vi "Get Enum Strings.vi"(8 "error in (no error)":errorcluster, 9 "Units":bool, 10 "Type":bool) -> (0 "error out":errorcluster, 1 "Units":cluster{"String":string, "Value":u16}[](array[cluster]), 2 "Type":cluster{"String":string, "Value":u16}[](array[cluster]))   [LabVIEW 2017, in "Modules.lvlib" / "9213.lvclass"]
uses:
  9213.lvclass
  Thermocouple Type.ctl
  Measurement Units.ctl
panel:
  out "Measurement Units":T1 items=["Raw Volts", "Degrees Kelvin", "Degrees Celsius", "Degrees Fahrenheit", "Degrees Rankine"]
  out "Thermocouple Type":T2 items=["J", "K", "T", "E", "R", "S", "N", "B"]
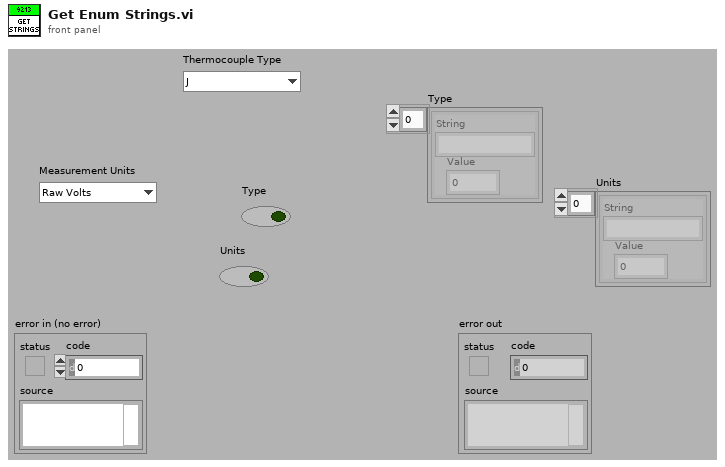
[diagram p1: front panel]
types:
  T1 = typedef "Modules.lvlib/9213.lvclass/Measurement Units.ctl" = u8
  T2 = typedef "Modules.lvlib/9213.lvclass/Thermocouple Type.ctl" = u8
  T3 = typedef "LVStringsAndValuesArrayTypeDef_U8.ctl" = cluster{"String":string, "Value":u8}[]
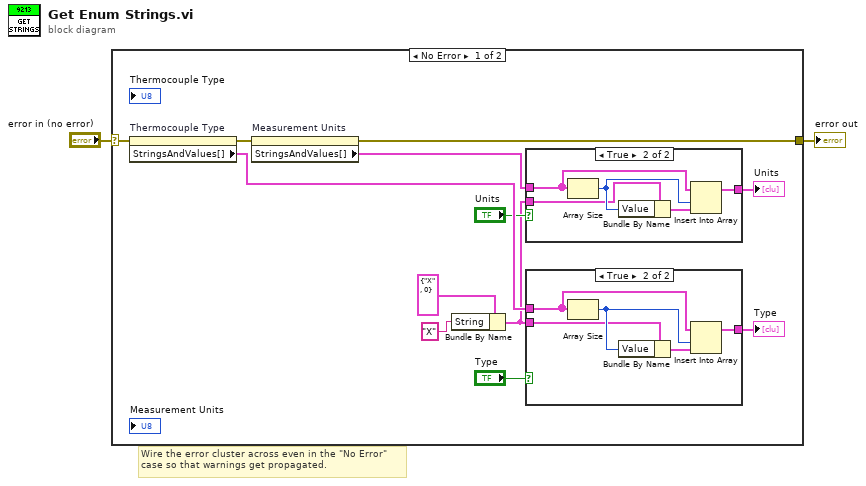
[diagram p0: block diagram]
diagram:
  # "Wire the error cluster across even in the \"No Error\"\ncase so that warnings get propagated."
  n1 = case shown="No Error" "error in (no error)" {
    selector: "error in (no error)" -> [w6 w27]
    tunnel: [w4 w27] -> w1
    frame No Error {
      n2 = property on="Thermocouple Type" class="Ring (strict)"(error in=w6) -> (error out=w5:errorcluster, "StringsAndValues[]"=w13:T3)  [unwired: 1 in, 1 out]
      n3 = property on="Measurement Units" class="Ring (strict)"(error in=w5) -> (error out=w4:errorcluster, "StringsAndValues[]"=w9:T3)  [unwired: 1 in, 1 out]
      n4 = Bundle By Name(cluster=cluster{"String":string, "Value":u16} {"String"="X", "Value"=0}, "String"="X") -> (w7:cluster{"String":string, "Value":u16})
      n5 = case shown="True" "Units" {
        tunnel: w9 -> [w15 w20]
        tunnel: [w15 w19] -> w10
        tunnel: w7 -> [_ w16]
        frame False {
        }
        frame True {
          n6 = Array Size(array=w20) -> (size(s)=w17:i32)
          n7 = Bundle By Name(cluster=w16, "Value"=w17) -> (w18:cluster{"String":string, "Value":u16})
          n8 = Insert Into Array(array=w20, index=w17, new element=w18) -> (w19:T3)
        }
      }
      "Units" <- w10
      n9 = case shown="True" "Type" {
        tunnel: w13 -> [w21 w26]
        tunnel: [w21 w25] -> w12
        tunnel: w7 -> [_ w22]
        frame False {
        }
        frame True {
          n10 = Array Size(array=w26) -> (size(s)=w23:i32)
          n11 = Bundle By Name(cluster=w22, "Value"=w23) -> (w24:cluster{"String":string, "Value":u16})
          n12 = Insert Into Array(array=w26, index=w23, new element=w24) -> (w25:T3)
        }
      }
      "Type" <- w12
    }
    frame Error {
    }
  }
  "error out" <- w1
